vi "Locate Spark.vi"(5 "Channel Data":dbl[][](array[numeric]), 9 "Correlation Window Offset (S)":dbl=0.0006, 11 "Correlation Window Duration (S)":dbl=0.0006, 12 "Sensor Locations (cm, cm, cm)":dbl[][](array[numeric])=[[0.0, 0.0, -0.04048], [0.1143, 0.0, 0.0], [0.0, 0.1143, 0.0], [-0.1143, 0.0, 0.0], [0.0, -0.1143, 0.0], [0.0, 0.0, 0.04048]]) -> (8 "Coordinates (cm, rad, cm)":cluster{sgl, sgl, sgl})   [LabVIEW 2013]
panel:
  # "x"
  # "y"
  # "z"
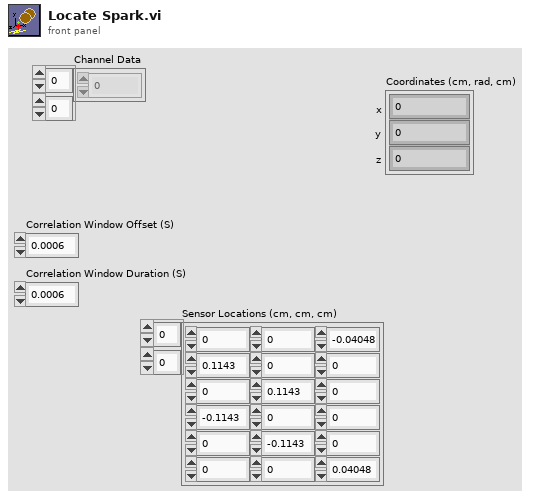
[diagram p1: front panel]
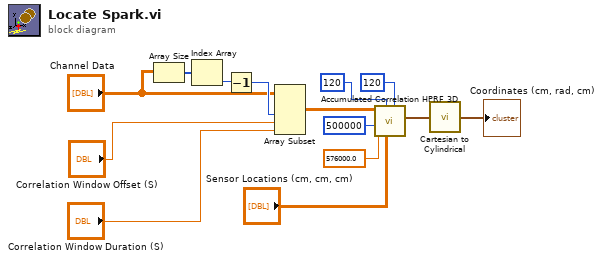
[diagram p0: block diagram]
diagram:
  n1 = Array Size(array="Channel Data") -> (size(s)=w11:i32[])
  n2 = Index Array(array=w11) -> (element=w10:i32)  [unwired: 1 in]
  n3 = Decrement(x=w10) -> (x-1=w9:i32)
  n4 = Array Subset(array="Channel Data", length (row)=w9, index (col)="Correlation Window Offset (S)", length (col)="Correlation Window Duration (S)") -> (w8:dbl[][])  [unwired: 1 in]
  n5 = call "Accumulated Correlation HPRF 3D.vi"("Ntheta"=120, "Sensor Locations (cm, cm, cm)"="Sensor Locations (cm, cm, cm)", "Nr"=120, "Sound Velocity (cm/s)"=576000.0, "Sampling Rate"=500000, "Waveforms"=w8) -> ("Coordinates (cm, cm, cm)"=w2:cluster{"x":dbl, "y":dbl, "z":dbl})  [unwired: 5 in]
  n6 = call "Cartesian to Cylindrical.vi"("Cartesian\nCoordinates"=w2) -> ("Cylindrical\nCoordinates"=→"Coordinates (cm, rad, cm)":cluster{"r":dbl, "theta":dbl, "z":dbl})  [unwired: 4 in]
